vi "DAQNavi Write (Digital 1D Wfm NChan 1Samp).vi"(8 "error in (no error)":errorcluster, 9 "timeout":dbl=10.0, 10 "data":digitalwaveform[](array[waveform]), 11 "task in":i32) -> (0 "error out":errorcluster, 2 "number of samples written per channel":u32, 3 "task out":i32)   [LabVIEW 2020]
uses:
  <vilib>/Waveform/DWDTOps.llb/DWDT Digital to Binary U8.vi
  DAQNavi_LV.dll
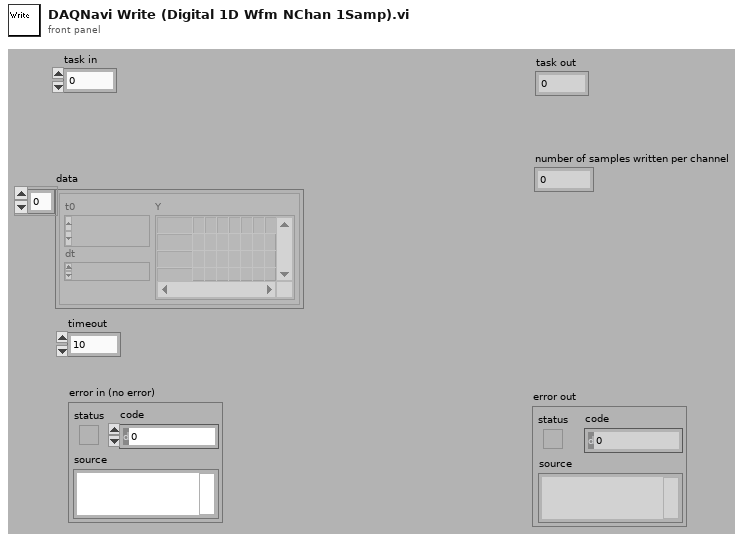
[diagram p1: front panel]
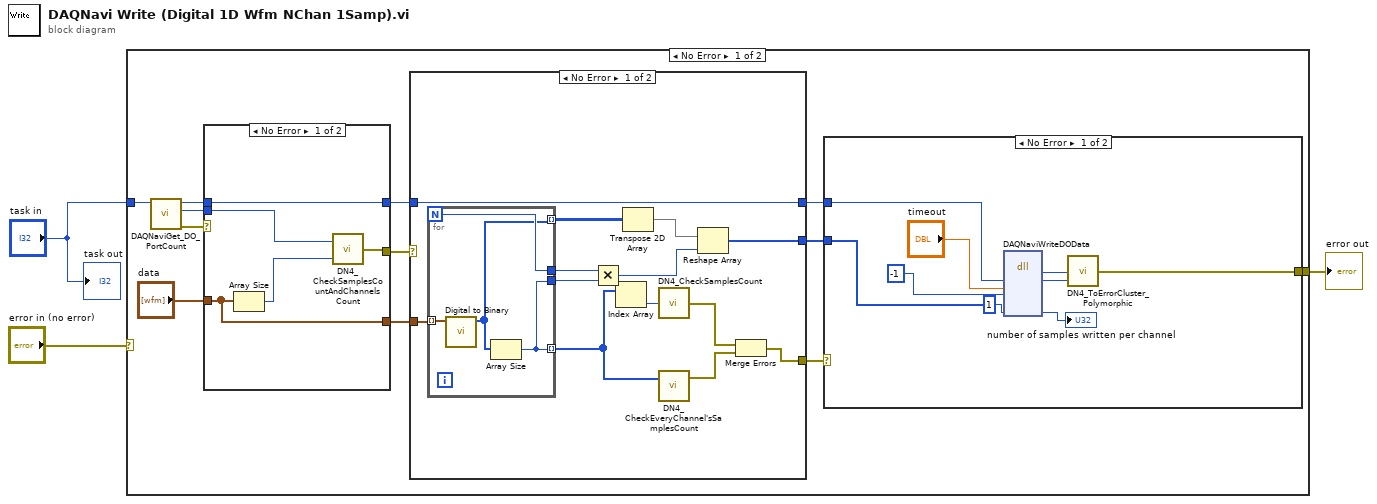
[diagram p0: block diagram]
diagram:
  n1 = case shown="No Error" "error in (no error)" {
    selector: "error in (no error)" -> [_ w53]
    tunnel: [w11 w53] -> w2
    tunnel: "task in" -> [w12 _]
    frame No Error {
      n2 = call "DAQNaviGet_DO_PortCount.vi"("task in"=w12) -> ("error out"=w15:errorcluster, "port count"=w14:i32, "task out"=w13:i32)  [unwired: 1 in, 7 out]
      n3 = case shown="No Error" w15 {
        selector: w15 -> [_ w42]
        tunnel: w14 -> [w37 _]
        tunnel: [w35 w42] -> w10
        tunnel: [w39 w41] -> w7
        tunnel: w13 -> [w39 w41]
        tunnel: "data" -> [w38 w40]
        tunnel: [w38 w40] -> w9
        frame No Error {
          n4 = Array Size(array=w38) -> (size(s)=w36:i32)
          n5 = call "DN4_CheckSamplesCountAndChannelsCount.vi"("samples count"=w36, "channel count"=w37) -> ("error out"=w35:errorcluster)
        }
        frame Error {
        }
      }
      n6 = case shown="No Error" w10 {
        selector: w10 -> [_ w34]
        tunnel: w9 -> [w28 _]
        tunnel: [w23 w34] -> w8
        tunnel: [w20 w33] -> w6
        tunnel: w7 -> [w20 w33]
        tunnel: [w19 _] -> w5
        frame No Error {
          n7 = for {
            N -> [w31]
            tunnel: w28 -> [w30] mode=indexing
            tunnel: [w32] -> w27 mode=indexing
            tunnel: [w29] -> w21 mode=indexing
            tunnel: [w32] -> w18
            tunnel: [w31] -> w17
            n8 = call-poly <vilib>:"Digital to Binary.vi"("digital waveform"=w30) -> ("binary array"=w29:u8[])  [unwired: 1 in, 9 out]
            n9 = Array Size(array=w29) -> (size(s)=w32:i32)
          }
          n10 = Multiply(x=w17, y=w18) -> (x*y=w16:i32)
          n11 = Index Array(array=w27) -> (element=w26:i32)  [unwired: 1 in]
          n12 = Transpose 2D Array(2D array=w21) -> (transposed array=w22:u8[][])
          n13 = call "DN4_CheckSamplesCount.vi"("samples count"=w26) -> ("error out"=w25:errorcluster)
          n14 = call "DN4_CheckEveryChannel'sSamplesCount.vi"("samples count"=w27) -> ("error out"=w24:errorcluster)  [unwired: 1 in]
          n15 = Reshape Array(w22, w16) -> (w19:u8[])
          n16 = Merge Errors(w25, w24) -> (w23:errorcluster)
        }
        frame Error {
        }
      }
      n17 = case shown="No Error" w8 {
        selector: w8 -> [_ w52]
        tunnel: [w51 w52] -> w11
        tunnel: w6 -> [w46 _]
        tunnel: w5 -> [w45 _]
        frame No Error {
          n18 = dll-call lib="DAQNavi_LV.dll" fn="DAQNaviWriteDOData"("taskID"=w46, "timeout"="timeout", "portBit"=-1, "portData"=w45, "samples"=u32 1) -> ("return type"=w48:i32, "taskID"=w44:i32, "samples"=→"number of samples written per channel":u32)  [unwired: 6 in, 2 out]
          n19 = call "DN4_ToErrorCluster_Polymorphic.vi"("task id"=w44, "error code"=w48) -> ("error out"=w51:errorcluster)  [unwired: 3 out]
        }
        frame Error {
        }
      }
    }
    frame Error {
    }
  }
  "error out" <- w2
  "task out" <- "task in"
